vi "Actor Core.vi"(8 "error in":errorcluster, 11 "WebSocket Connection in":refnum<class "WebSocket Connection.lvclass">) -> (0 "error out":errorcluster, 3 "Actor out":refnum<class "Actor.lvclass">)   [LabVIEW 2016, in "WebSocket Actor.lvlib" / "WebSocket Connection.lvclass"]
doc: "(<B>Filename</B>: Actor Framework.lvlib:Actor.lvclass:Actor Core.vi)\n\nReceives messages to the actor, reacts to them, and initiates any error handling that may shut the actor down.\n\nDescendant classes may override this VI to append parallel tasks for the actor to complete while it handles messages. Overrides use the Call Parent Method node."
uses:
  WebSocket Connection.lvclass
  C:/Program Files (x86)/National Instruments/LabVIEW 2016/vi.lib/ActorFramework/Actor/Actor.lvclass
  <vilib>/ActorFramework/Actor/Actor.lvclass
  <vilib>/ActorFramework/Actor/Actor.lvclass/Actor.ctl
  WebSocket Connection.lvclass/WebSocket Connection.ctl
  <vilib>/MediaMongrels Ltd/WebSockets/WebSockets/WebSockets.lvlib
  WebSocket Service Actor Messages/Transmit Data to Subscriber Msg/Transmit Data to Subscriber Msg.lvclass
panel:
  out "Received Data":string
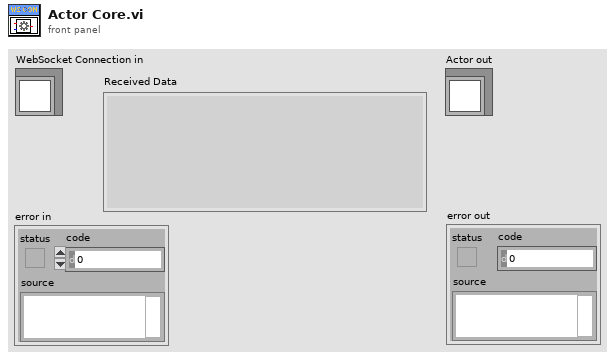
[diagram p1: front panel]
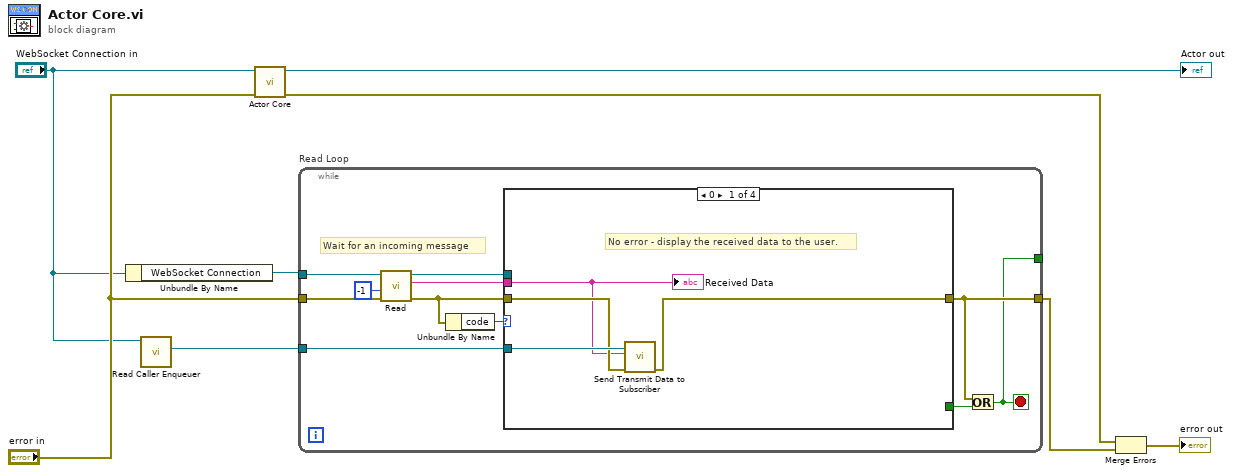
[diagram p0: block diagram]
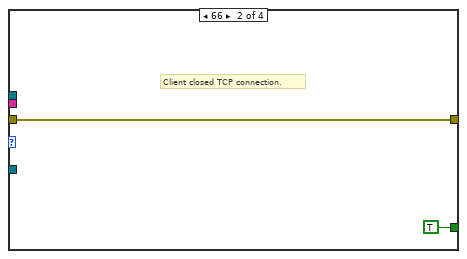
[diagram p2: hidden frame]
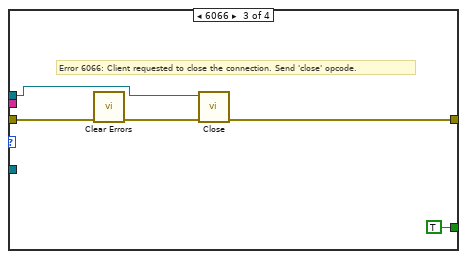
[diagram p3: hidden frame]
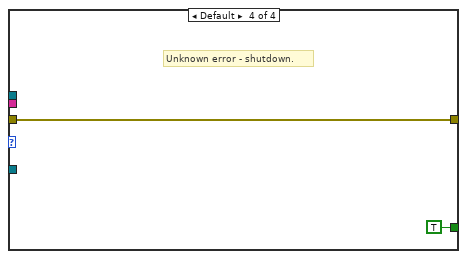
[diagram p4: hidden frame]
diagram:
  n1 = Unbundle By Name("WebSocket Connection in") -> ("WebSocket Connection"=w6:refnum<k5>)
  n2 = call <vilib>:"Read Caller Enqueuer.vi"("Actor"="WebSocket Connection in") -> ("Caller Enqueuer"=w1:refnum<class "Message Enqueuer.lvclass">)  [unwired: 10 in]
  n3 = call-parent "Actor Core.vi"("error in"="error in", "Actor in"="WebSocket Connection in") -> ("error out"=w8:errorcluster, "Actor out"=→"Actor out":refnum<class "Actor.lvclass">)  [unwired: 8 in]
  n4 = while "Read Loop" {
    tunnel: w6 -> [w19]
    tunnel: [w10] -> _
    tunnel: [w12] -> w3
    tunnel: "error in" -> [w13]
    tunnel: w1 -> [w9]
    stop <- w10 stop-if-true
    # "Wait for an incoming message"
    n5 = call <vilib>:"Read.vi"("error in (no error)"=w13, "timeout ms (5000)"=-1 ("timeout ms (25000)"), "WebSocket Connection in"=w19) -> ("error out"=w14:errorcluster, "Data"=w16:string, "WebSocket Connection out"=w15:refnum<k5>)  [unwired: 5 in, 1 out]
    n6 = Unbundle By Name(w14) -> ("code"=w17:i32)
    n7 = case shown="0" w17 {
      tunnel: w16 -> [w20 _ _ _]
      tunnel: [_ TRUE TRUE TRUE] -> w11
      tunnel: w15 -> [_ _ w30 _]
      tunnel: w14 -> [w22 w24 w28 w31]
      tunnel: [w21 w24 w27 w31] -> w12
      tunnel: w9 -> [w23 _ _ _]
      frame 0 {
        # "No error - display the received data to the user."
        n8 = call "Send Transmit Data to Subscriber.vi"("error in (no error)"=w22, "Received Data"=w20, "Message Enqueuer in"=w23) -> ("error out"=w21:errorcluster)  [unwired: 7 in, 1 out]
        "Received Data" <- w20
      }
      frame 66 {
        # "Client closed TCP connection."
      }
      frame 6066 {
        # "Error 6066: Client requested to close the connection. Send 'close' opcode."
        n9 = call <vilib>:"Clear Errors.vi"("error in (no error)"=w28) -> ("error out"=w26:errorcluster)  [unwired: 5 in, 1 out]
        n10 = call <vilib>:"Close.vi"("error in (no error)"=w26, "WebSocket Connection in"=w30) -> ("error out"=w27:errorcluster)  [unwired: 8 in, 1 out]
      }
      frame Default {
        # "Unknown error - shutdown."
      }
    }
    n11 = Or(x=w12, y=w11) -> (x .or. y?=w10:bool)
  }
  n12 = Merge Errors(w8, w3) -> (→"error out":errorcluster)
